vi "Write Data.vi"(5 "CS (None)":refnum<class "SPI CS.lvclass">, 7 "SPI":refnum<class "SPI.lvclass">, 8 "error in (no error)":errorcluster, 10 "Data":string, 11 "Session In":refnum<class "Session.lvclass">) -> (0 "error out":errorcluster, 3 "Session Out":refnum<class "Session.lvclass">)   [LabVIEW 2024, in "CTI.lvlib" / "SPI.lvclass"]
uses:
  SPI.lvclass
  SPI CS/SPI CS.lvclass
  Session/Session.lvclass
  SPI.lvclass/SPI.ctl
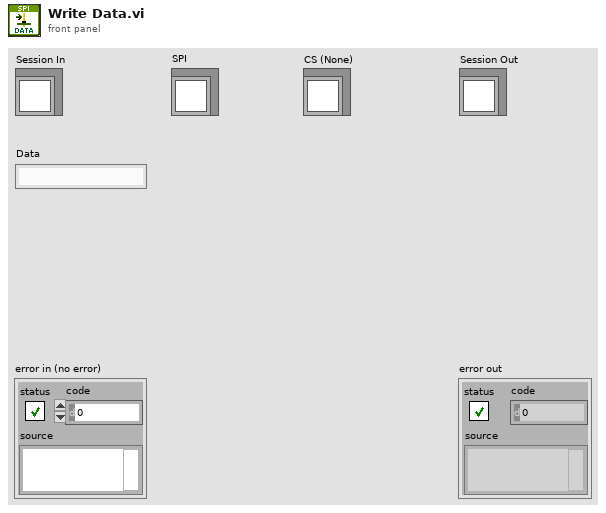
[diagram p1: front panel]
types:
  T1 = typedef "CTI.lvlib/SPI Number.ctl" = i8
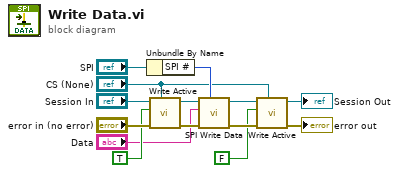
[diagram p0: block diagram]
diagram:
  n1 = Unbundle By Name("SPI") -> ("SPI #"=w6:T1)
  n2 = call "Write Active.vi"("SPI CS"="CS (None)", "error in (no error)"="error in (no error)", "Active"=TRUE, "Session In"="Session In") -> ("error out"=w10:errorcluster, "Session Out"=w8:refnum<class "Session.lvclass">)  [unwired: 6 in]
  n3 = call "SPI Write Data.vi"("SPI #"=w6, "error in (no error)"=w10, "Data"="Data", "Session in"=w8) -> ("error out"=w13:errorcluster, "Session out"=w9:refnum<class "Session.lvclass">)  [unwired: 6 in]
  n4 = call "Write Active.vi"("SPI CS"="CS (None)", "error in (no error)"=w13, "Active"=FALSE, "Session In"=w9) -> ("error out"=→"error out":errorcluster, "Session Out"=→"Session Out":refnum<class "Session.lvclass">)  [unwired: 6 in]
